vi "Get PPS Terminal Default.vi"(11 "TimeKeeper Module":string) -> (3 "PPSTerminal Default":string)   [LabVIEW 2019, in "NI Synchronization System Explorer.lvlib"]
uses:
  NI Synchronization System Explorer.lvlib
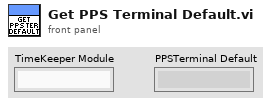
[diagram p1: front panel]
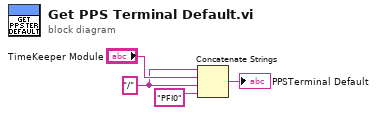
[diagram p0: block diagram]
diagram:
  w1 = "/" ("string")
  n1 = Concatenate Strings(w1, "TimeKeeper Module", w1, "PFI0" ("string")) -> (→"PPSTerminal Default":string)
